vi "Test - Licence Check.vi"(8 "error in":errorcluster, 11 "licence key (optional)":string) -> (0 "error out":errorcluster, 2 "options":variant, 3 "licence key":string)   [LabVIEW 2013]
uses:
  <vilib>/ErrorRing/Error Ring.xnode
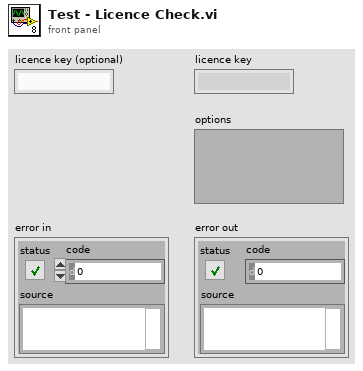
[diagram p1: front panel]
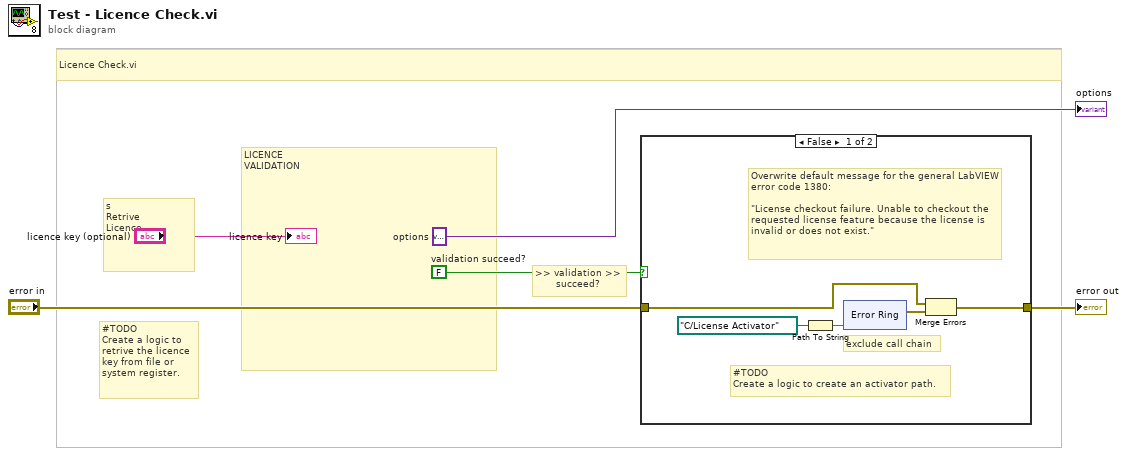
[diagram p0: block diagram]
diagram:
  w2 = variant  # options
  w4 = FALSE  # validation succeed?
  # "#TODO\nCreate a logic to retrive the licence key from file or system register."
  # "s\nRetrive\nLicence"
  # "LICENCE\nVALIDATION"
  # "Licence Check.vi"
  # ">> validation >>\n       succeed?"
  n1 = case shown="False" w4 {
    tunnel: [w7 w16] -> w5
    tunnel: "error in" -> [w6 w16]
    frame False {
      # "#TODO\nCreate a logic to create an activator path."
      # "Overwrite default message for the general LabVIEW error code 1380:\n\n\"License checkout failure. Unable to checkout the requested license feature because the license is invalid or does not exist.\""
      # "exclude call chain"
      n2 = Path To String(path=path "C:/License Activator") -> (string=w9:string)
      n3 = xnode "Error Ring"("parameter 0"=w9) -> ("error out"=w8:errorcluster)
      n4 = Merge Errors(w6, w8) -> (w7:errorcluster)
    }
    frame True {
    }
  }
  "error out" <- w5
  "options" <- w2
  "licence key" <- "licence key (optional)"
